vi "plot focus curve.vi"(8 "error in (no error)":errorcluster, 11 "Autofocus in":refnum<class "Autofocus.lvclass">) -> (0 "error out":errorcluster, 1 "x array":dbl[](array[numeric]), 2 "y array":dbl[](array[numeric]), 3 "Autofocus out":refnum<class "Autofocus.lvclass">)   [LabVIEW 2012, in "Autofocus.lvclass"]
uses:
  Autofocus.lvclass
  Autofocus.lvclass/Autofocus.ctl
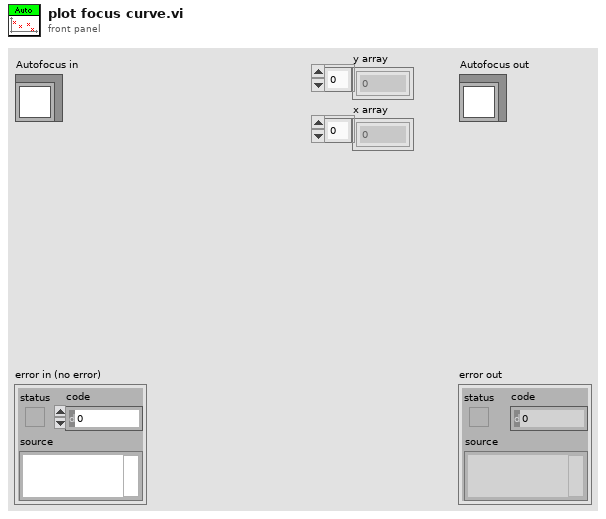
[diagram p1: front panel]
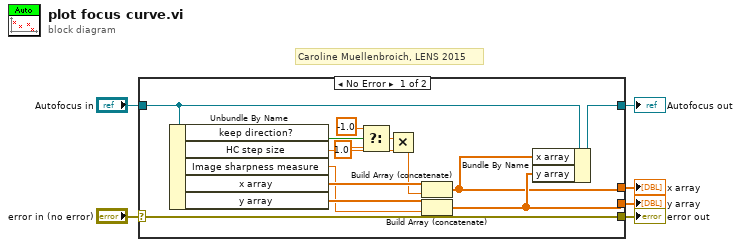
[diagram p0: block diagram]
diagram:
  # "Caroline Muellenbroich, LENS 2015"
  n1 = case shown="No Error" "error in (no error)" {
    selector: "error in (no error)" -> [w20 w22]
    tunnel: [w20 w22] -> w5
    tunnel: [w13 w21] -> w3
    tunnel: "Autofocus in" -> [w14 w21]
    tunnel: [w8 _] -> w2
    tunnel: [w7 _] -> w1
    frame No Error {
      n2 = Unbundle By Name(w14) -> ("keep direction?"=w17:bool, "HC step size"=w15:dbl, "Image sharpness measure"=w9:dbl, "x array"=w12:dbl[], "y array"=w10:dbl[])
      n3 = Select(t=-1.0 ("y"), s=w17, f=1.0 ("y")) -> (s? t:f=w16:dbl)
      n4 = Multiply(x=w16, y=w15) -> (x*y=w11:dbl)
      n5 = Build Array (concatenate)(w12, w11) -> (w7:dbl[])
      n6 = Build Array (concatenate)(w10, w9) -> (w8:dbl[])
      n7 = Bundle By Name(cluster=w14, "x array"=w7, "y array"=w8) -> (w13:refnum<class "Autofocus.lvclass">)
    }
    frame Error {
    }
  }
  "error out" <- w5
  "Autofocus out" <- w3
  "y array" <- w2
  "x array" <- w1
